vi "MGCC_StaEst_pinv.vi"(1 "G3":dbl[][](array[numeric])) -> (0 "Ginv":dbl[][](array[numeric]))   [LabVIEW 2016]
uses:
  <vilib>/imath/engines/lvmath2/RunTimeEngine/BuiltInFunctions/pinv/NIMS_pinv.vi
  <instcachedir>/0/NIMS_pinv_206F0700CF75499C820074BA4F1FFC36.lvgen/NIMS_pinv_206F0700CF75499C820074BA4F1FFC36_000.vi
  <vilib>/imath/engines/lvmath2/RunTimeEngine/ErrorHandling/NIMS_Error From Error Code.vi
  <vilib>/imath/engines/lvmath2/RunTimeEngine/NodeEndStatement/NIMS_NodeEndStatement_Output.vi
  <instcachedir>/0/NIMS_NodeEndStatement_Output_53EC0D466D134D7ABD903AC30B43404B.lvgen/NIMS_NodeEndStatement_Output_53EC0D466D134D7ABD903AC30B43404B_002.vi
  <vilib>/imath/engines/lvmath2/RunTimeEngine/ErrorHandling/NIMS_Finalize Error.vi
panel:
  out "error out":errorcluster
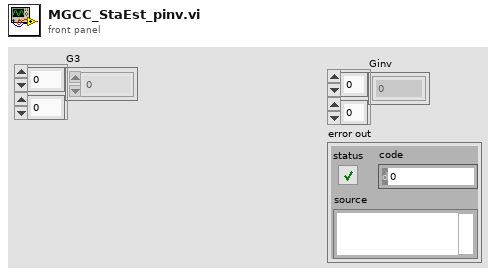
[diagram p1: front panel]
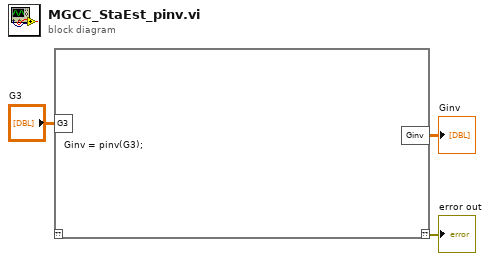
[diagram p0: block diagram]
diagram:
  n1 = mathscript code="Ginv = pinv(G3);"("G3"="G3") -> ("??"=→"error out":errorcluster, "Ginv"=→"Ginv":dbl[][])  [unwired: 1 in]
